vi "create.open.paths.vi"(6 "disable buffering (F)":bool, 8 "error in":errorcluster) -> (0 "error out":errorcluster, 2 "binary references":T1, 3 "output cluster":T2={"volumes path"=path "", "issues path"=path "", "publishers path"=path "D:/Comics/data/cv_issues"})   [LabVIEW 2024, in "manager_daemon.lvclass"]
uses:
  manager_daemon.lvclass
  type_defs/paths--cluster.ctl
  binary.references--cluster.ctl
  manager_daemon.lvclass/manager_daemon.ctl
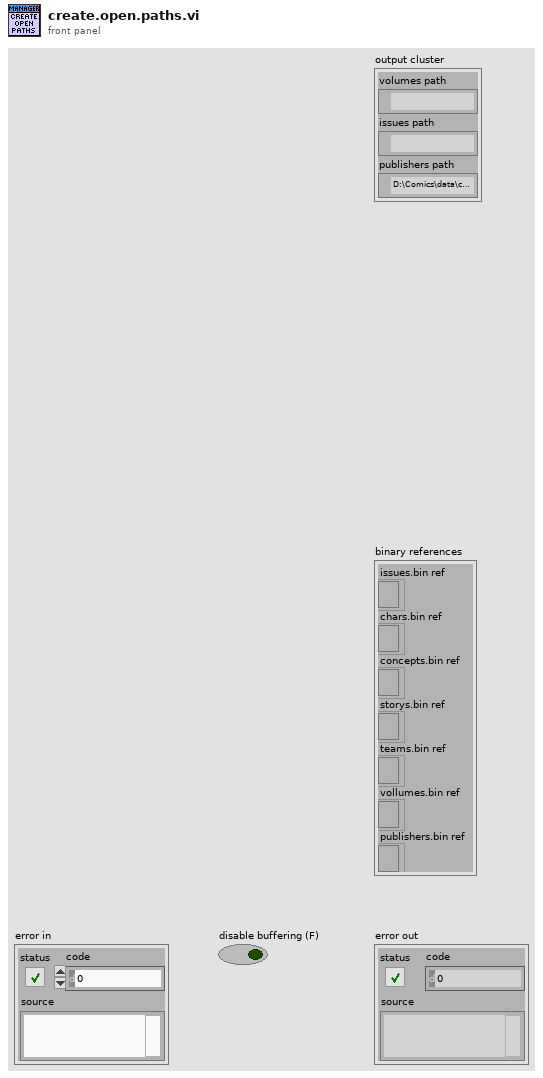
[diagram p1: front panel]
types:
  T1 = typedef "manager_daemon.lvclass/binary.references--cluster.ctl" = cluster{"issues.bin ref":refnum<file>, "chars.bin ref":refnum<file>, "concepts.bin ref":refnum<file>, "storys.bin ref":refnum<file>, "teams.bin ref":refnum<file>, "vollumes.bin ref":refnum<file>, "publishers.bin ref":refnum<file>}
  T2 = typedef "manager_daemon.lvclass/paths--cluster.ctl" = cluster{"volumes path":path, "issues path":path, "publishers path":path}
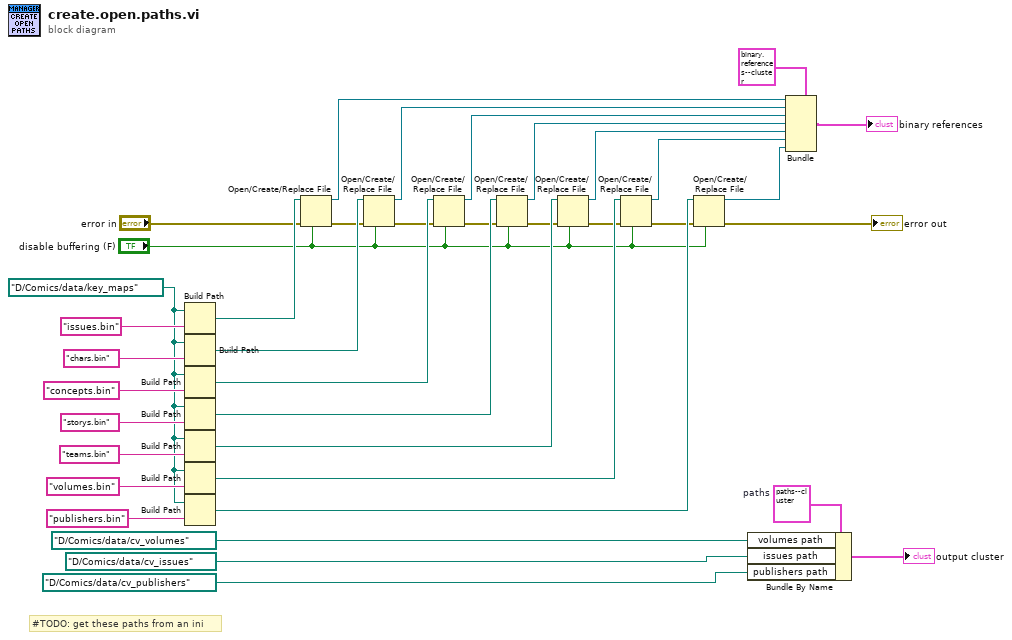
[diagram p0: block diagram]
diagram:
  w29 = path "D:/Comics/data/key_maps" ("issue map path")
  w38 = T2 {"volumes path"=path "", "issues path"=path "", "publishers path"=path "D:/Comics/data/cv_issues"}  # paths
  # "#TODO: get these paths from an ini"
  n1 = Build Path(base path=w29, name or relative path="issues.bin") -> (appended path=w27:path)
  n2 = Build Path(base path=w29, name or relative path="chars.bin") -> (appended path=w26:path)
  n3 = Build Path(base path=w29, name or relative path="concepts.bin") -> (appended path=w25:path)
  n4 = Build Path(base path=w29, name or relative path="storys.bin") -> (appended path=w24:path)
  n5 = Build Path(base path=w29, name or relative path="teams.bin") -> (appended path=w23:path)
  n6 = Build Path(base path=w29, name or relative path="volumes.bin") -> (appended path=w22:path)
  n7 = Build Path(base path=w29, name or relative path="publishers.bin") -> (appended path=w20:path)
  n8 = Open/Create/Replace File(file path (use dialog)=w27, error in="error in", disable buffering (F)="disable buffering (F)") -> (refnum out=w9:refnum<file>, error out=w18:errorcluster)  [unwired: 3 in, 1 out]
  n9 = Open/Create/Replace File(file path (use dialog)=w26, error in=w18, disable buffering (F)="disable buffering (F)") -> (refnum out=w8:refnum<file>, error out=w17:errorcluster)  [unwired: 3 in, 1 out]
  n10 = Open/Create/Replace File(file path (use dialog)=w25, error in=w17, disable buffering (F)="disable buffering (F)") -> (refnum out=w7:refnum<file>, error out=w16:errorcluster)  [unwired: 3 in, 1 out]
  n11 = Open/Create/Replace File(file path (use dialog)=w24, error in=w16, disable buffering (F)="disable buffering (F)") -> (refnum out=w6:refnum<file>, error out=w15:errorcluster)  [unwired: 3 in, 1 out]
  n12 = Open/Create/Replace File(file path (use dialog)=w23, error in=w15, disable buffering (F)="disable buffering (F)") -> (refnum out=w5:refnum<file>, error out=w14:errorcluster)  [unwired: 3 in, 1 out]
  n13 = Open/Create/Replace File(file path (use dialog)=w22, error in=w14, disable buffering (F)="disable buffering (F)") -> (refnum out=w4:refnum<file>, error out=w13:errorcluster)  [unwired: 3 in, 1 out]
  n14 = Open/Create/Replace File(file path (use dialog)=w20, error in=w13, disable buffering (F)="disable buffering (F)") -> (refnum out=w3:refnum<file>, error out=→"error out":errorcluster)  [unwired: 3 in, 1 out]
  n15 = Bundle By Name(cluster=w38, "volumes path"=path "D:/Comics/data/cv_volumes" ("issue map path"), "issues path"=path "D:/Comics/data/cv_issues" ("issue map path"), "publishers path"=path "D:/Comics/data/cv_publishers" ("issue map path")) -> (→"output cluster":T2)
  n16 = Bundle(cluster=T1 {"issues.bin ref"=refnum, "chars.bin ref"=refnum, "concepts.bin ref"=refnum, "storys.bin ref"=refnum, "teams.bin ref"=refnum, "vollumes.bin ref"=refnum, "publishers.bin ref"=refnum} ("binary references"), "issues.bin ref"=w9, "chars.bin ref"=w8, "concepts.bin ref"=w7, "storys.bin ref"=w6, "teams.bin ref"=w5, "vollumes.bin ref"=w4, "publishers.bin ref"=w3) -> (→"binary references":T1)
